vi "!_Read-Write_Setups.vi"(2 "Port Settings Array In":T1[](array[typedef]) {"flow control etc."."parity err byte" format="%.0x"; "flow control etc."."XON byte" format="%.0x"; "flow control etc."."XOFF byte" format="%.0x"; "data bits" min=5 max=8 step=1}, 3 "Setup Name":string, 4 "Mode":enum16{"Load serial setup", "Save serial setup"}(ring)) -> (0 "Port Settings Array Out":T1[](array[typedef]) {"flow control etc."."parity err byte" format="%.0x"; "flow control etc."."XON byte" format="%.0x"; "flow control etc."."XOFF byte" format="%.0x"; "data bits" min=5 max=8 step=1}, 1 "error unflattening":bool)   [LabVIEW 2016]
uses:
  Port_Params.ctl
  Anemometry/Anemometry Sub Vis/Globals/Constants_global.vi
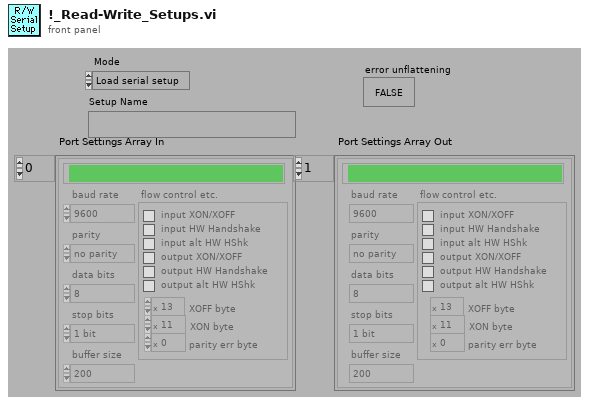
[diagram p1: front panel]
types:
  T1 = typedef "Port_Params.ctl" = cluster{"Name":string, "flow control etc.":cluster{"input XON/XOFF":bool, "input HW Handshake":bool, "input alt HW HShk":bool, "output XON/XOFF":bool, "output HW Handshake":bool, "output alt HW HShk":bool, "XOFF byte ":u8, "XON byte":u8, "parity err byte":u16}, "buffer size":u16, "baud rate":u32, "data bits":u16, "stop bits":enum16{"1 bit", "1.5 bits", "2 bits"}, "parity":enum16{"no parity", "odd parity", "even parity", "mark parity", "space parity"}}
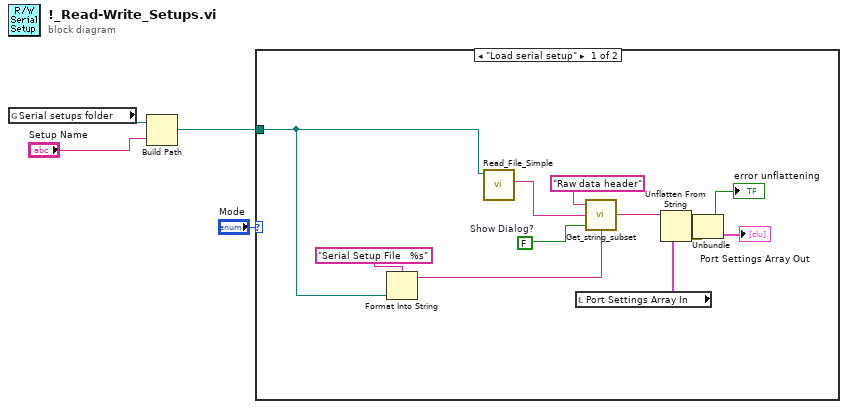
[diagram p0: block diagram]
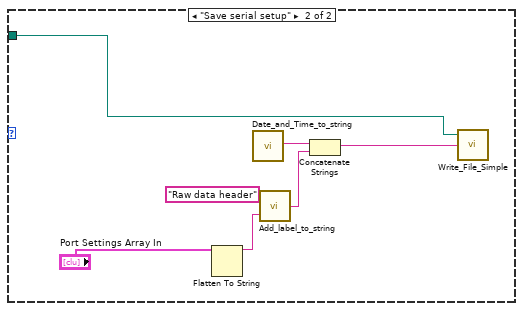
[diagram p2: hidden frame]
diagram:
  n1 = global read "Constants_global.vi" "Serial setups folder"() -> (w3:path)
  n2 = Build Path(base path=w3, name or relative path="Setup Name") -> (appended path=w2:path)
  n3 = case shown="\"Load serial setup\"" "Mode" {
    tunnel: w2 -> [w5 w17]
    frame "Load serial setup" {
      w11 = FALSE  # Show Dialog?
      n4 = Format Into String(format string="Serial Setup File   %s", w5) -> (resulting string=w6:string)  [unwired: 2 in, 1 out]
      n5 = call "Read_File_Simple.vi"("Filename"=w5) -> ("string"=w14:string)  [unwired: 2 in, 7 out]
      n6 = local read "Port Settings Array In"() -> (w9:T1[])
      n7 = call "Get_string_subset.vi"("String Name"=w6, "Show Dialog?"=w11, "String to split"=w14, "File Label"="Raw data header") -> ("Output string"=w13:string)  [unwired: 1 out]
      n8 = Unflatten From String(type=w9, binary string=w13) -> (value=→"Port Settings Array Out":T1[], error out=w8:errorcluster)  [unwired: 1 in, 3 out]
      n9 = Unbundle(w8) -> ("status"=→"error unflattening":bool)  [unwired: 2 out]
    }
    frame "Save serial setup" {
      n10 = Flatten To String(anything="Port Settings Array In") -> (data string=w22:string)  [unwired: 1 in, 4 out]
      n11 = call "Date_and_Time_to_string.vi"() -> ("Date and time (spreadsheet)"=w20:string)
      n12 = call "Add_label_to_string.vi"("String to write"=w22, "File Label"="Raw data header") -> ("Output string"=w19:string)
      n13 = Concatenate Strings(w20, w19) -> (w16:string)
      n14 = call "Write_File_Simple.vi"("character string"=w16, "file path"=w17) -> ()  [unwired: 1 in, 2 out]
    }
  }
